vi "BPM-Chassis01 FPGA.vi"() -> ()   [LabVIEW 2010]
uses:
  <vilib>/eio/EIONode/EIONode.xnode
  <vilib>/rvi/eio/nirviEIOImplementation/nirviEIOImplementation.xnode
  <vilib>/rvi/eio/common/nirviEmuClasses.ctl
  <vilib>/eio/EIOMethodNode/EIOMethodNode.xnode
  <vilib>/rvi/eio/nirviEIOMethodImplementation/nirviEIOMethodImplementation.xnode
  <vilib>/rvi/Analysis/measure/butterworth/XNode/niFpgaButterworthFilter.xnode
  <vilib>/rvi/eio/common/nirviEmuTemplateMethod_noerrors.vi
panel:
  out "Mod3/AI3":fxp<+/-,20,5> format="%.17g"
  out "Mod3/AI2":fxp<+/-,20,5> format="%.17g"
  out "Mod1/AI1":fxp<+/-,20,5> format="%.17g"
  out "Mod2/AI3":fxp<+/-,20,5> format="%.17g"
  out "Mod2/AI2":fxp<+/-,20,5> format="%.17g"
  out "Mod2/AI1":fxp<+/-,20,5> format="%.17g"
  out "Mod2/AI0":fxp<+/-,20,5> format="%.17g"
  out "Mod1/AI3":fxp<+/-,20,5> format="%.17g"
  out "Mod1/AI2":fxp<+/-,20,5> format="%.17g"
  out "Mod1/AI0":fxp<+/-,20,5> format="%.17g"
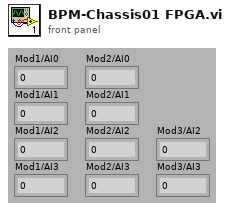
[diagram p1: front panel]
types:
  T1 = typedef "nirviEmuClasses.ctl" = enum16{"IO Read", "IO Write", "Method", "Property Read", "Property Write"}
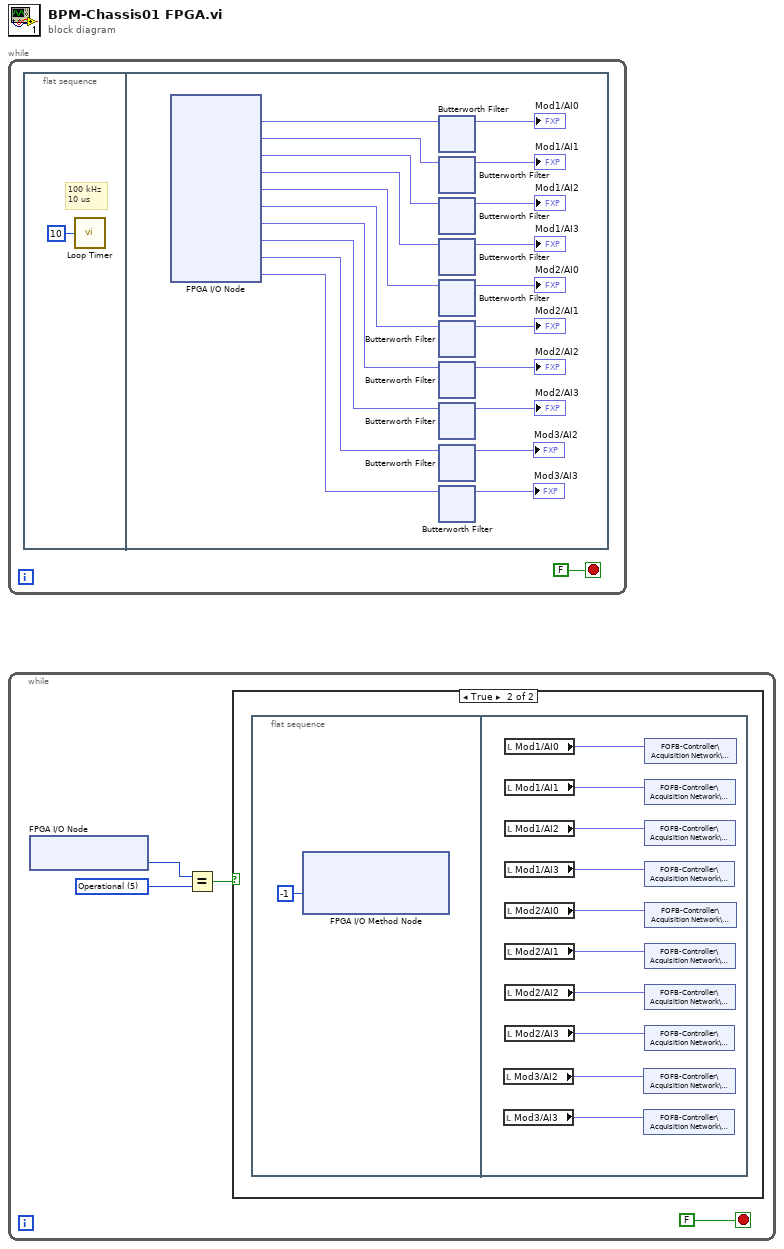
[diagram p0: block diagram]
diagram:
  n1 = while {
    stop <- FALSE stop-if-true
    n2 = flat-sequence {
      frame #0 {
        # "100 kHz\n10 us"
        n3 = call "Loop Timer"("Count(uSec)"=u8 10) -> ()  [unwired: 1 out]
      }
      frame #1 {
        n4 = xnode "FPGA I/O Node"() -> ("Mod1/AI0"=w22:fxp<+/-,20,5>, "Mod1/AI1"=w18:fxp<+/-,20,5>, "Mod1/AI2"=w17:fxp<+/-,20,5>, "Mod1/AI3"=w16:fxp<+/-,20,5>, "Mod2/AI0"=w15:fxp<+/-,20,5>, "Mod2/AI1"=w14:fxp<+/-,20,5>, "Mod2/AI2"=w13:fxp<+/-,20,5>, "Mod2/AI3"=w20:fxp<+/-,20,5>, "Mod3/AI2"=w6:fxp<+/-,20,5>, "Mod3/AI3"=w5:fxp<+/-,20,5>)  [unwired: 10 in, 10 out]
        n5 = xnode "Butterworth Filter"("input data"=w22) -> ("output data"=→"Mod1/AI0":fxp<+/-,20,5>)  [unwired: 2 in]
        n6 = xnode "Butterworth Filter"("input data"=w18) -> ("output data"=→"Mod1/AI1":fxp<+/-,20,5>)  [unwired: 2 in]
        n7 = xnode "Butterworth Filter"("input data"=w17) -> ("output data"=→"Mod1/AI2":fxp<+/-,20,5>)  [unwired: 2 in]
        n8 = xnode "Butterworth Filter"("input data"=w16) -> ("output data"=→"Mod1/AI3":fxp<+/-,20,5>)  [unwired: 2 in]
        n9 = xnode "Butterworth Filter"("input data"=w15) -> ("output data"=→"Mod2/AI0":fxp<+/-,20,5>)  [unwired: 2 in]
        n10 = xnode "Butterworth Filter"("input data"=w14) -> ("output data"=→"Mod2/AI1":fxp<+/-,20,5>)  [unwired: 2 in]
        n11 = xnode "Butterworth Filter"("input data"=w13) -> ("output data"=→"Mod2/AI2":fxp<+/-,20,5>)  [unwired: 2 in]
        n12 = xnode "Butterworth Filter"("input data"=w20) -> ("output data"=→"Mod2/AI3":fxp<+/-,20,5>)  [unwired: 2 in]
        n13 = xnode "Butterworth Filter"("input data"=w6) -> ("output data"=→"Mod3/AI2":fxp<+/-,20,5>)  [unwired: 2 in]
        n14 = xnode "Butterworth Filter"("input data"=w5) -> ("output data"=→"Mod3/AI3":fxp<+/-,20,5>)  [unwired: 2 in]
      }
    }
  }
  n15 = while {
    stop <- FALSE stop-if-true
    w307 = u8 5 items=["Init"=1, "PreOp"=2, "Bootstrap"=3, "SafeOp"=4, "Operational"=5]
    n16 = xnode "FPGA I/O Node"() -> ("EtherCAT State"=w306:u8)  [unwired: 1 in, 1 out]
    n17 = Equal?(x=w306, y=w307) -> (x = y?=w305:bool)
    n18 = case shown="True" w305 {
      frame False {
      }
      frame True {
        n19 = flat-sequence {
          frame #0 {
            n20 = xnode "FPGA I/O Method Node"("Timeout"=-1) -> ()  [unwired: 1 in, 2 out]
          }
          frame #1 {
            n21 = local read "Mod3/AI2"() -> (w333:fxp<+/-,20,5>)
            n22 = local read "Mod3/AI3"() -> (w334:fxp<+/-,20,5>)
            n23 = local read "Mod1/AI0"() -> (w342:fxp<+/-,20,5>)
            n24 = local read "Mod1/AI1"() -> (w341:fxp<+/-,20,5>)
            n25 = local read "Mod1/AI2"() -> (w340:fxp<+/-,20,5>)
            n26 = local read "Mod1/AI3"() -> (w339:fxp<+/-,20,5>)
            n27 = local read "Mod2/AI0"() -> (w338:fxp<+/-,20,5>)
            n28 = local read "Mod2/AI1"() -> (w337:fxp<+/-,20,5>)
            n29 = local read "Mod2/AI2"() -> (w336:fxp<+/-,20,5>)
            n30 = local read "Mod2/AI3"() -> (w335:fxp<+/-,20,5>)
            n31 = shared-variable "FOFB-Controller\\Acquisition Network\\BPM-Chassis01\\User-Defined Variables\\AMP03CH"(w333) -> ()  [unwired: 1 in, 1 out]
            n32 = shared-variable "FOFB-Controller\\Acquisition Network\\BPM-Chassis01\\User-Defined Variables\\AMP03CV"(w334) -> ()  [unwired: 1 in, 1 out]
            n33 = shared-variable "FOFB-Controller\\Acquisition Network\\BPM-Chassis01\\User-Defined Variables\\AMP02AH"(w342) -> ()  [unwired: 1 in, 1 out]
            n34 = shared-variable "FOFB-Controller\\Acquisition Network\\BPM-Chassis01\\User-Defined Variables\\AMP02AV"(w341) -> ()  [unwired: 1 in, 1 out]
            n35 = shared-variable "FOFB-Controller\\Acquisition Network\\BPM-Chassis01\\User-Defined Variables\\AMP02BH"(w340) -> ()  [unwired: 1 in, 1 out]
            n36 = shared-variable "FOFB-Controller\\Acquisition Network\\BPM-Chassis01\\User-Defined Variables\\AMP02BV"(w339) -> ()  [unwired: 1 in, 1 out]
            n37 = shared-variable "FOFB-Controller\\Acquisition Network\\BPM-Chassis01\\User-Defined Variables\\AMP03AH"(w338) -> ()  [unwired: 1 in, 1 out]
            n38 = shared-variable "FOFB-Controller\\Acquisition Network\\BPM-Chassis01\\User-Defined Variables\\AMP03AV"(w337) -> ()  [unwired: 1 in, 1 out]
            n39 = shared-variable "FOFB-Controller\\Acquisition Network\\BPM-Chassis01\\User-Defined Variables\\AMP03BH"(w336) -> ()  [unwired: 1 in, 1 out]
            n40 = shared-variable "FOFB-Controller\\Acquisition Network\\BPM-Chassis01\\User-Defined Variables\\AMP03BV"(w335) -> ()  [unwired: 1 in, 1 out]
          }
        }
      }
    }
  }
